vi "Create Instrument.vi"(8 "error in (no error)":errorcluster, 9 "Debug Mode? [F]":bool, 10 "Configuration Window? [T]":bool=TRUE, 11 "Instrument in":refnum<class "Instrument.lvclass">) -> (0 "error out":errorcluster, 3 "Instrument out":refnum<class "Instrument.lvclass">)   [LabVIEW 2016, in "Instrument.lvclass"]
uses:
  Instrument.lvclass
  C:/Program Files (x86)/National Instruments/LabVIEW 2016/vi.lib/JKI/JKI SMO/SMO/SMO.lvclass
  Instrument.lvclass/Instrument.ctl
  <vilib>/JKI/JKI SMO/SMO/SMO.lvclass
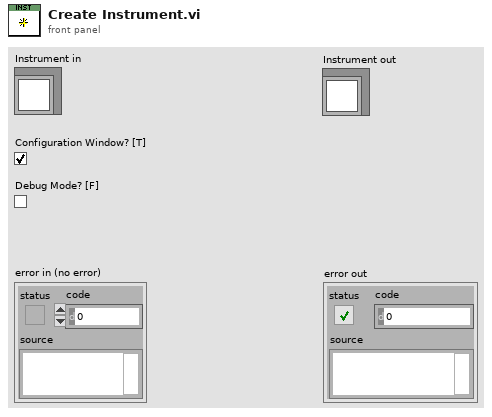
[diagram p1: front panel]
types:
  T1 = typedef "Instrument.lvclass/SMO RC Type--enum.ctl" = enum16{"RC", "STM", "ZMQ"}
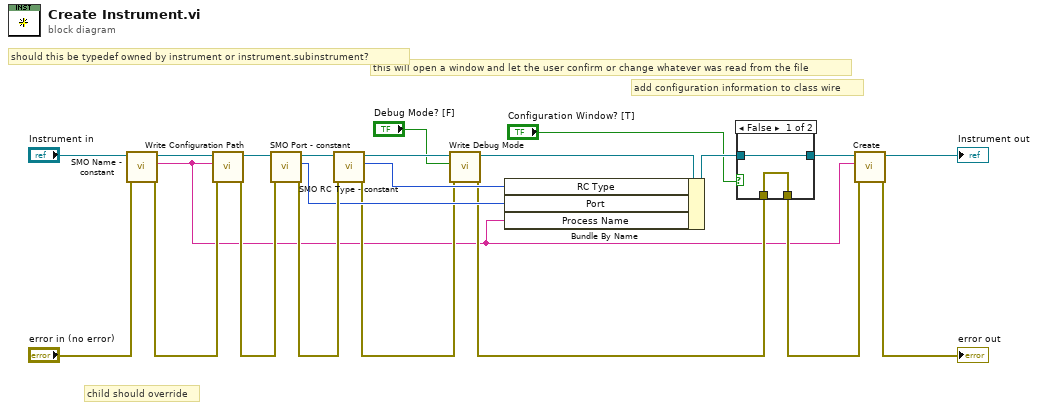
[diagram p0: block diagram]
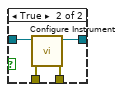
[diagram p2: hidden frame]
diagram:
  # "this will open a window and let the user confirm or change whatever was read from the file"
  # "child should override"
  # "add configuration information to class wire"
  # "should this be typedef owned by instrument or instrument.subinstrument?"
  n1 = call-dynamic "SMO Name - constant.vi"("error in (no error)"="error in (no error)", "Instrument in"="Instrument in") -> ("error out"=w18:errorcluster, "SMO Name"=w1:string, "Instrument out"=w16:refnum<class "Instrument.lvclass">)  [unwired: 7 in]
  n2 = call "Write Configuration Path.vi"("error in (no error)"=w18, "name or relative path"=w1, "Instrument in"=w16) -> ("error out"=w13:errorcluster, "Instrument out"=w14:refnum<class "Instrument.lvclass">)  [unwired: 7 in]
  n3 = call-dynamic "SMO Port - constant.vi"("error in (no error)"=w13, "Instrument in"=w14) -> ("error out"=w10:errorcluster, "Port"=w9:u16, "Instrument out"=w15:refnum<class "Instrument.lvclass">)  [unwired: 7 in]
  n4 = call-dynamic "SMO RC Type - constant.vi"("error in (no error)"=w10, "Instrument in"=w15) -> ("error out"=w4:errorcluster, "Configuration.SMO.RC Type"=w11:T1, "Instrument out"=w7:refnum<class "Instrument.lvclass">)  [unwired: 7 in]
  n5 = call "Write Debug Mode.vi"("error in (no error)"=w4, "Debug Mode?"="Debug Mode? [F]", "Instrument in"=w7) -> ("error out"=w3:errorcluster, "Instrument out"=w6:refnum<class "Instrument.lvclass">)  [unwired: 7 in]
  n6 = Bundle By Name(cluster=w6, "RC Type"=w11, "Port"=w9, "Process Name"=w1) -> (w8:refnum<class "Instrument.lvclass">)
  n7 = case shown="False" "Configuration Window? [T]" {
    tunnel: [w23 w28] -> w17
    tunnel: [w24 w27] -> w12
    tunnel: w8 -> [w24 w26]
    tunnel: w3 -> [w23 w25]
    frame False {
    }
    frame True {
      n8 = call-dynamic "Configure Instrument.vi"("error in (no error)"=w25, "Instrument in"=w26) -> ("error out"=w28:errorcluster, "Instrument out"=w27:refnum<class "Instrument.lvclass">)  [unwired: 8 in]
    }
  }
  n9 = call <vilib>:"Create.vi"("error in (no error)"=w17, "Subsystem Name (optional)"=w1, "SMO"=w12) -> ("error out"=→"error out":errorcluster, "SMO out"=→"Instrument out":refnum<class "Instrument.lvclass">)  [unwired: 6 in, 1 out]
